vi "Read Action.vi"(11 "ActionStack in":refnum<class "Action.lvclass">) -> (2 "Action":string, 3 "ActionStack out":refnum<class "Action.lvclass">)   [LabVIEW 2024, in "ActionStack.lvlib" / "Action.lvclass"]
uses:
  Action.lvclass
  Action.lvclass/Action.ctl
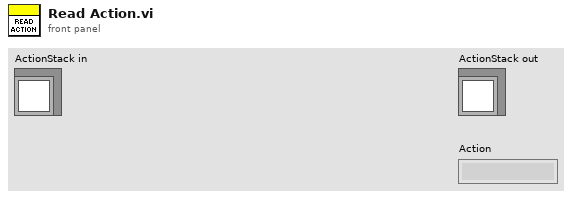
[diagram p1: front panel]
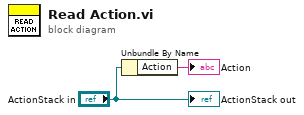
[diagram p0: block diagram]
diagram:
  n1 = Unbundle By Name("ActionStack in") -> ("Action"=→"Action":string)
  "ActionStack out" <- "ActionStack in"
